vi "ClusterUnderstandingProperly.vi"() -> ()   [LabVIEW 2019]
panel:
  out "Are you Married  Or Not":bool
  out "Your Full Name":string
  out "Your Age":dbl
  in  "Cluster":T1
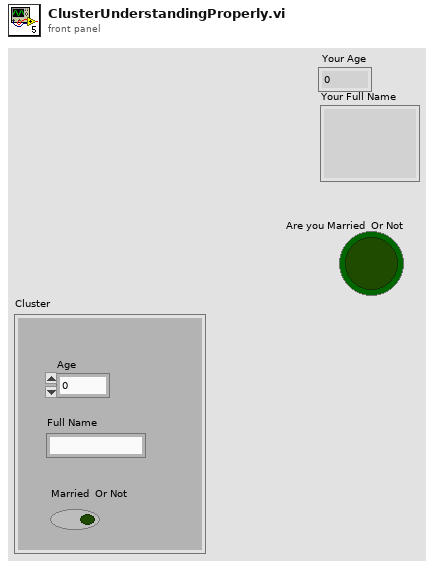
[diagram p1: front panel]
types:
  T1 = cluster{"Age":dbl, "Full Name ":string, "Married  Or Not ":bool}
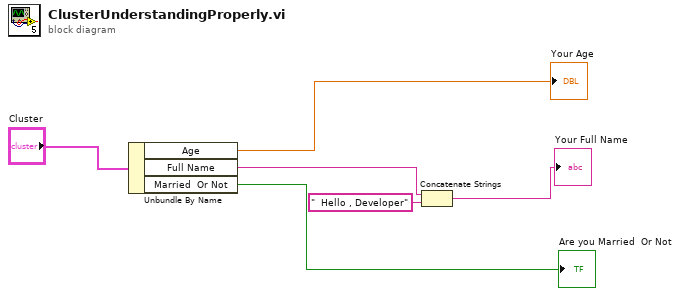
[diagram p0: block diagram]
diagram:
  n1 = Unbundle By Name("Cluster") -> ("Age"=→"Your Age":dbl, "Full Name"=w3:string, "Married  Or Not"=→"Are you Married  Or Not":bool)
  n2 = Concatenate Strings(w3, "  Hello , Developer" ("string")) -> (→"Your Full Name":string)
